vi "User_Current_Write.vi"(6 "User_Remember_Name":bool, 7 "User_Remember_PW":bool, 8 "error in (no error)":errorcluster caption="错误输入（无错误）", 9 "Password":string, 10 "User_Right":u16(ring) caption="权    限" items=["管理员", "操作员"], 11 "Name":string) -> (0 "error out":errorcluster caption="错误输出")   [LabVIEW 2020]
uses:
  <vilib>/addons/database/NI_Database_API.lvlib
  <vilib>/drjdpowell/SQLite Library/SQL Connection/Connection.lvclass
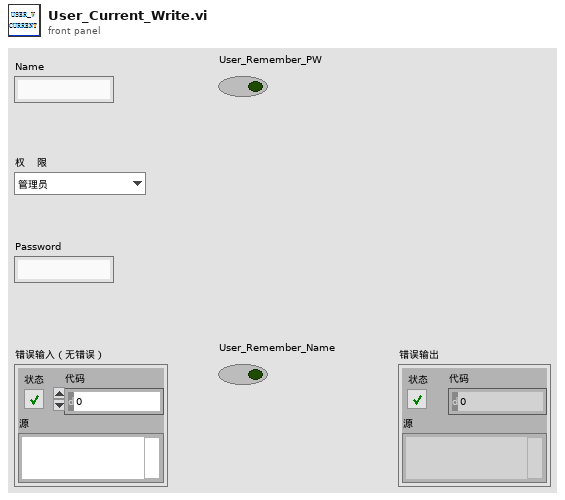
[diagram p1: front panel]
types:
  T1 = cluster{"Name":string, "output string":string, "Password":string, "User_Remember_Name":bool, "User_Remember_PW":bool}
  T2 = cluster{"Name":string, "output string":string, "Password":string}
  T3 = typedef "NI_Database_API.lvlib/Conn ObjectReference.ctl" = refnum<k1>
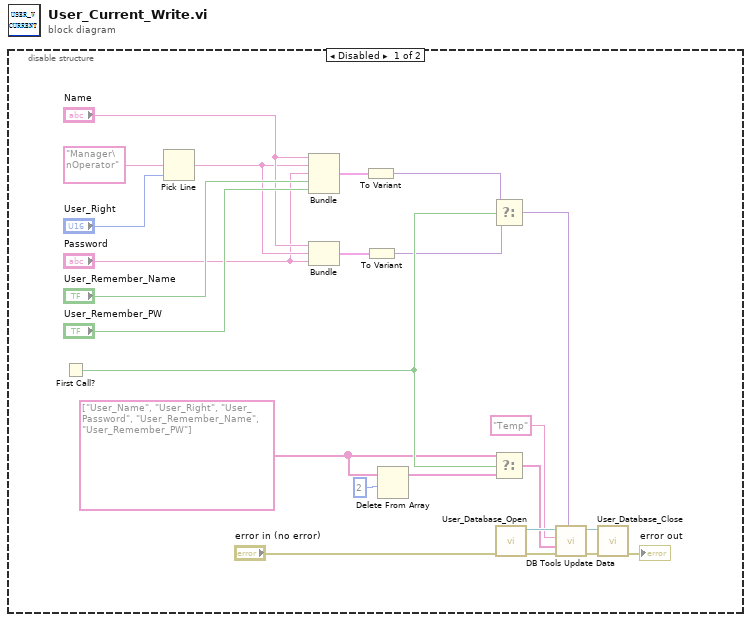
[diagram p0: block diagram]
diagram:
  n1 = disable-structure shown="Disabled" {
    frame Disabled {
      w6 = string[] ["User_Name", "User_Right", "User_Password", "User_Remember_Name", "User_Remember_PW"]
      n2 = First Call?() -> (First Call?: T/F=w7:bool)
      n3 = Pick Line(multi-line string="Manager\nOperator" ("多行字符串"), line index="User_Right") -> (output string=w10:string)  [unwired: 1 in]
      n4 = Bundle("Name"="Name", "output string"=w10, "Password"="Password", "User_Remember_Name"="User_Remember_Name", "User_Remember_PW"="User_Remember_PW") -> (w13:T1)  [unwired: 1 in]
      n5 = Bundle("Name"="Name", "output string"=w10, "Password"="Password") -> (w8:T2)  [unwired: 1 in]
      n6 = To Variant(anything=w13) -> (Variant=w12:variant)
      n7 = To Variant(anything=w8) -> (Variant=w1:variant)
      n8 = Delete From Array(array=w6, length=2 ("长度")) -> (array with subset deleted=w4:string[])  [unwired: 1 in, 1 out]
      n9 = Select(t=w12, s=w7, f=w1) -> (s? t:f=w2:variant)
      n10 = Select(t=w6, s=w7, f=w4) -> (s? t:f=w3:string[])
      n11 = call "User_Database_Open.vi"("error in (no error)"="error in (no error)") -> ("error out"=w21:errorcluster, "SQLite Connection"=w22:refnum<class "Connection.lvclass">)  [unwired: 9 in]
      n12 = call <vilib>:"DB Tools Update Data.vi"("data"=w2, "error in (no error)"=w21, "columns"=w3, "table"="Temp", "connection reference"=w22) -> ("error out"=w19:errorcluster, "connection reference out"=w18:T3)  [unwired: 5 in]
      n13 = call "User_Database_Close.vi"("error in (no error)"=w19, "SQLite Connection in"=w18) -> ("error out"=→"error out":errorcluster)  [unwired: 9 in]
    }
    frame Enabled {
    }
  }
